vi "GoLocal.vi"(8 "LV ERROR IN":errorcluster, 11 "CONFIGURATION CLUSTER":T1) -> (0 "LV ERROR OUT":errorcluster)   [LabVIEW 2012]
doc: "Sets the AVS-47B in local mode\nand closes the VISA session. Terminate\nyour application always with this VI."
panel:
  # "GoLocal.vi"
  # "This VI should be used in the end of an application to close the open VISA session (another possibility\nis to set LabView to close VISA sessions automatically). Using this VI is, however better, because it \nleaves the AVS-47B in the local mode without changing any other settings. It is a good practise to leave \nthe bridge in local, when the application VI exits. Next time, the application can be started in local \nmode and the  existing settings can be safely read to be the initial values for the subsequent remote control.\nUnexpected changes in settings can be avoided this way.\n\nBe very careful in starting the remote mode in applications including the TS-530A\ntemperature controller. Because of its old design, its settings cannot be read, they can\nonly be controlled.  Be sure to set all the PID parameters in your application to safe values before \nstarting remote mode."
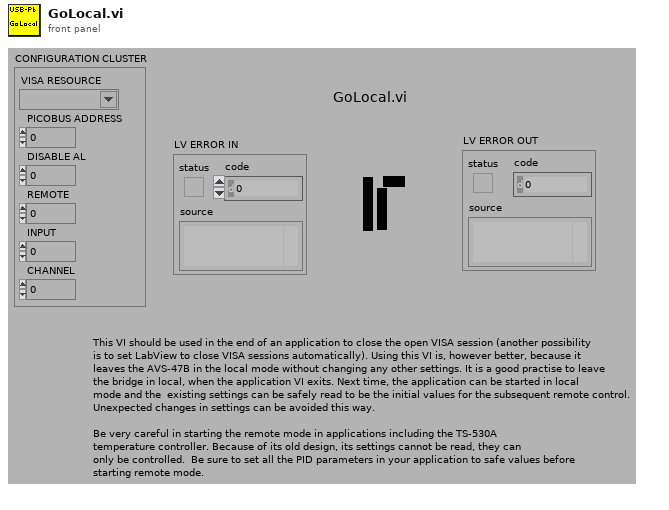
[diagram p1: front panel]
types:
  T1 = cluster{"VISA RESOURCE":refnum<visa-resource-name>, "PICOBUS ADDRESS":u8, "DISABLE AL":u8, "REMOTE":u8, "INPUT":u8, "CHANNEL":u8, "RANGE":u8, "EXCITATION":u8, "DISPLAY":u8, "DIGITAL REFERENCE":u16, "SET POINT":dbl, "PROP GAIN":u8, "INTG":u8, "DERIV":u8, "POWER BIAS":u8, "POWER RANGE":u8, "INFO STRING":string, "HEATER RESISTANCE":dbl, "INTERVAL":u8, " SENSOR dR/dT":u8}
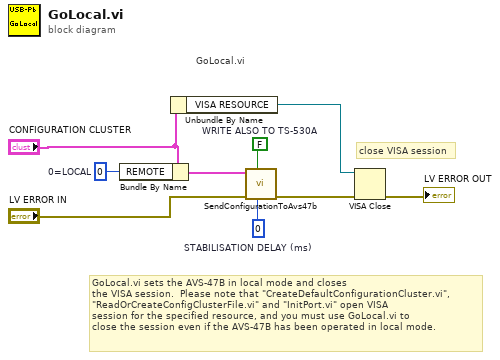
[diagram p0: block diagram]
diagram:
  w5 = 0  # STABILISATION DELAY (ms)
  w6 = FALSE  # WRITE ALSO TO TS-530A
  w9 = u8 0  # 0=LOCAL
  # "GoLocal.vi sets the AVS-47B in local mode and closes\nthe VISA session.  Please note that \"CreateDefaultConfigurationCluster.vi\",\n\"ReadOrCreateConfigClusterFile.vi\" and \"InitPort.vi\" open VISA\nsession for the specified resource, and you must use GoLocal.vi to\nclose the session even if the AVS-47B has been operated in local mode."
  # "GoLocal.vi"
  # "close VISA session"
  n1 = Bundle By Name(cluster="CONFIGURATION CLUSTER", "REMOTE"=w9) -> (w8:T1)
  n2 = Unbundle By Name("CONFIGURATION CLUSTER") -> ("VISA RESOURCE"=w3:refnum<visa-resource-name>)
  n3 = call "SendConfigurationToAvs47b.vi"("STABILISATION DELAY (ms)"=w5, "WRITE ALSO TO TS-530A"=w6, "LV ERROR IN"="LV ERROR IN", "CONFIGURATION CLUSTER"=w8) -> ("LV ERROR OUT"=w4:errorcluster)  [unwired: 4 in, 3 out]
  n4 = VISA Close(VISA resource name=w3, error in (no error)=w4) -> (error out=→"LV ERROR OUT":errorcluster)
